vi "Wait Until Next us Multiple.vi"(11 "Numeric":dbl) -> ()   [LabVIEW 2015]
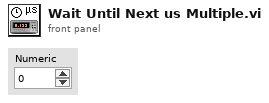
[diagram p1: front panel]
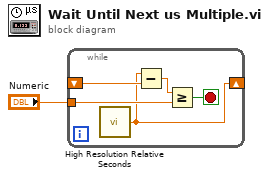
[diagram p0: block diagram]
diagram:
  n1 = while {
    tunnel: "Numeric" -> [w4]
    shift-right: [w2] -> _
    shift-left: _ -> [w6]
    stop <- w5 stop-if-true
    n2 = call <vilib>:"High Resolution Relative Seconds.vi"() -> ("relative seconds"=w2:dbl)
    n3 = Subtract(x=w2, y=w6) -> (x-y=w3:dbl)
    n4 = Greater Or Equal?(x=w3, y=w4) -> (x >= y?=w5:bool)
  }
